vi "Write Channels.vi"(10 "Channels":T1[](array[typedef]), 11 "NI USB-6501 in":refnum<class "NI USB-6501.lvclass">) -> (3 "NI USB-6501 out":refnum<class "NI USB-6501.lvclass">)   [LabVIEW 2020, in "NI USB-6501.lvclass"]
uses:
  NI USB-6501.lvclass
  Controls/Channel.ctl
  NI USB-6501.lvclass/NI USB-6501.ctl
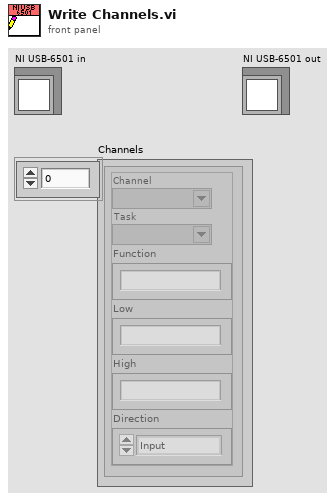
[diagram p1: front panel]
types:
  T1 = typedef "NI USB-6501.lvclass/Channel.ctl" = cluster{"Channel":tag, "Task":refnum<k21>, "Function":string, "Low":string, "High":string, "Direction":enum16{"Input", "Output"}}
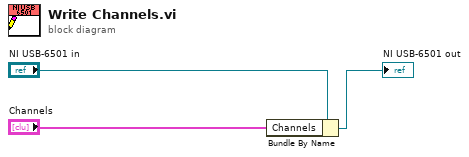
[diagram p0: block diagram]
diagram:
  n1 = Bundle By Name(cluster="NI USB-6501 in", "Channels"="Channels") -> (→"NI USB-6501 out":refnum<class "NI USB-6501.lvclass">)
